vi "ntr.status-table-init.vi"(8 "error IN":errorcluster, 11 "Table in":refnum<vi>) -> (0 "error out":errorcluster, 3 "Table out":refnum<vi>)   [LabVIEW 2024]
uses:
  <vilib>/Utility/miscctls.llb/LVRowAndColumnTypeDef.ctl
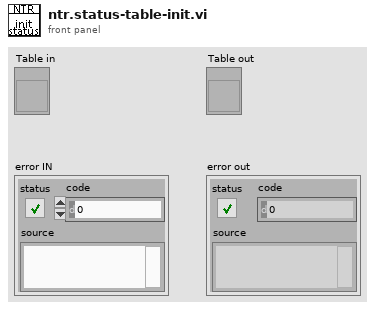
[diagram p1: front panel]
types:
  T1 = typedef "LVRowAndColumnTypeDef.ctl" = cluster{"Row":i32, "Column":i32}
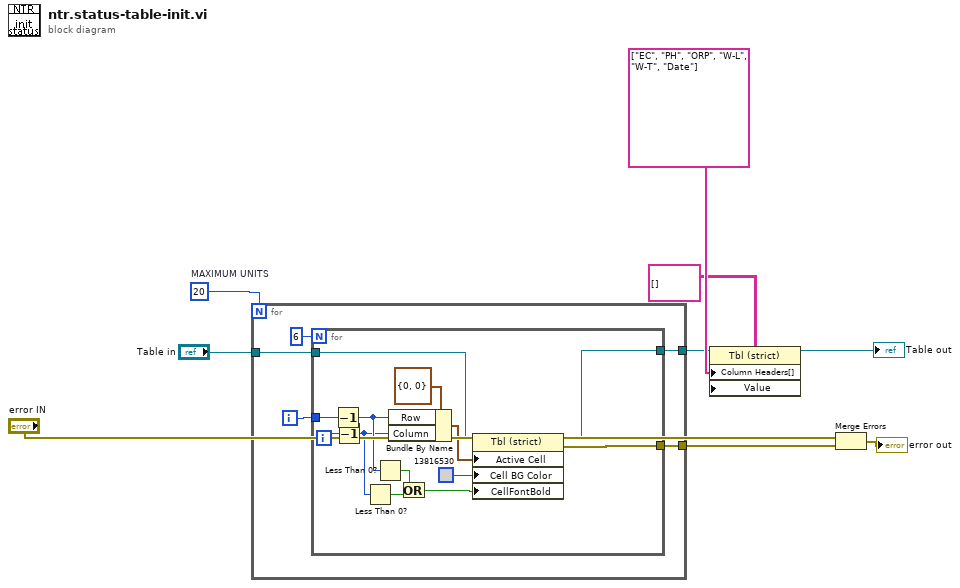
[diagram p0: block diagram]
diagram:
  w7 = 20  # MAXIMUM UNITS
  n1 = for {
    N: w7 -> [_]
    tunnel: "Table in" -> [w13]
    tunnel: [w12] -> w8
    tunnel: [w11] -> w5
    i -> [w14]
    n2 = for {
      N: 6 -> [_]
      tunnel: w14 -> [w26]
      tunnel: w13 -> [w23]
      tunnel: [w22] -> w12
      tunnel: [w15] -> w11
      i -> [w20]
      n3 = Decrement(x=w26) -> (x-1=w21:i32)
      n4 = Decrement(x=w20) -> (x-1=w16:i32)
      n5 = Less Than 0?(x=w16) -> (x < 0?=w18:bool)
      n6 = Less Than 0?(x=w21) -> (x < 0?=w19:bool)
      n7 = Bundle By Name(cluster=T1 {"Row"=0, "Column"=0} ("Active Cell:Active Cell"), "Row"=w21, "Column"=w16) -> (w24:T1)
      n8 = Or(x=w19, y=w18) -> (x .or. y?=w17:bool)
      n9 = property class="Tbl (strict)"(reference=w23, "Active Cell"=w24, "Cell BG Color"=u32 13816530, "CellFontBold"=w17) -> (reference out=w15:refnum<vi>, error out=w22:errorcluster)  [unwired: 1 in]
    }
  }
  n10 = property class="Tbl (strict)"(reference=w5, "Column Headers[]"=string[] ["EC", "PH", "ORP", "W-L", "W-T", "Date"], "Value"=string[][] []) -> (reference out=→"Table out":refnum<vi>)  [unwired: 1 in, 1 out]
  n11 = Merge Errors("error IN", w8) -> (→"error out":errorcluster)
